vi "KB-新画十字线.vi"(10 "数组":T2[](array[typedef]) {"Correlation Score" format="%.2f"; "Target Template Curve Score" format="%.2f"; "Template Target Curve Score" format="%.2f"; "Bounding Box"."y" format="%.2f"; "Bounding Box"."x" format="%.2f"; "Position"."y" format="%.2f"; "Position"."x" format="%.2f"; "Score" format="%.2f"; "Scale" format="%.2f"; "Angle" format="%.2f"; "Occlusion %" format="%.2f"}, 11 "输入图片":T1(plugin-control)) -> (2 "Position":cluster{"x":sgl, "y":sgl}, 3 "输出图片":T1(plugin-control))   [LabVIEW 2015]
uses:
  <vilib>/vision/Pattern Matching.llb/IMAQ GM Match Report.ctl
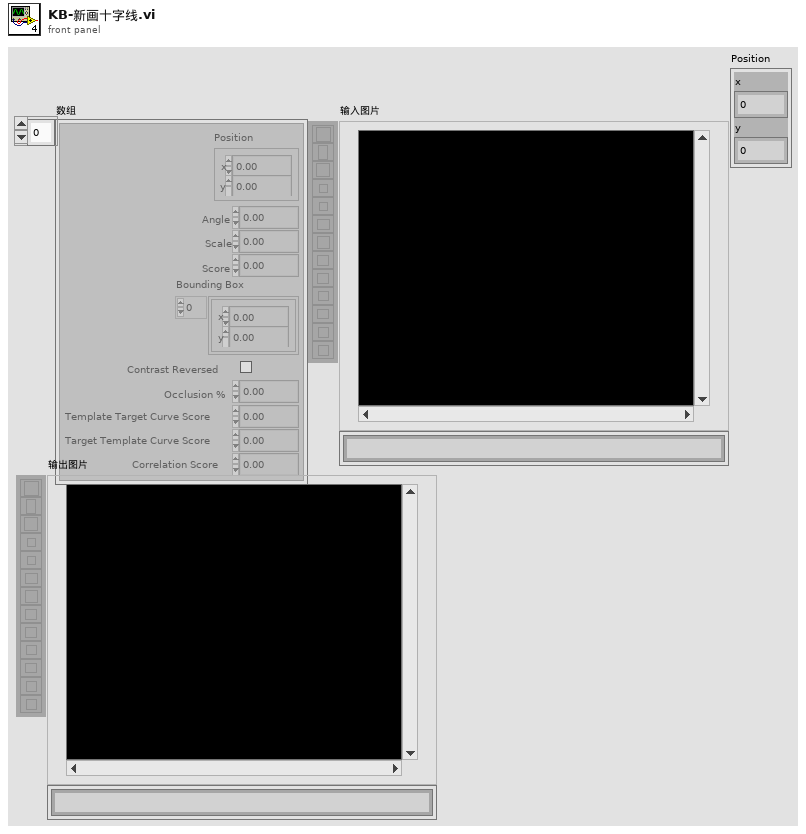
[diagram p1: front panel]
types:
  T1 = typedef "IMAQ Image.ctl" = refnum<image>
  T2 = typedef "IMAQ GM Match Report.ctl" = cluster{"Position":cluster{"x":sgl, "y":sgl}, "Angle":sgl, "Scale":sgl, "Score":sgl, "Bounding Box":cluster{"x":sgl, "y":sgl}[], "Contrast Reversed":bool, "Occlusion %":sgl, "Template Target Curve Score":sgl, "Target Template Curve Score":sgl, "Correlation Score":sgl}
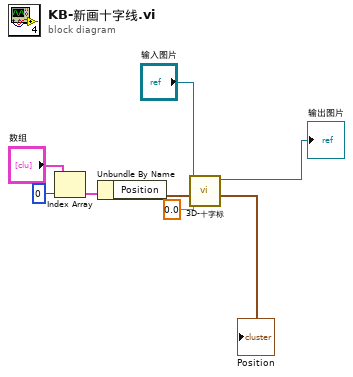
[diagram p0: block diagram]
diagram:
  n1 = Index Array(array="数组", index=0 ("索引")) -> (element=w3:T2)
  n2 = Unbundle By Name(w3) -> ("Position"=w7:cluster{"x":sgl, "y":sgl})
  "Position" <- w7
  n3 = call "3D-十字标.vi"("radius"=0.0, "CenterPos"=w7, "输入图片"="输入图片") -> ("输出图片"=→"输出图片":T1)  [unwired: 7 in, 1 out]
